vi "PH_BeamlineController.set PA DP Target GUI Elements.vi"(0 "VI in":refnum<vi>, 5 "error in (no error)":errorcluster) -> (14 "VI out":refnum<vi>, 19 "error out":errorcluster)   [LabVIEW 2014, in "PH_BeamlineController.lvlib"]
uses:
  PH_BeamlineController.lvlib
  PH_SystemInformation/PH_SystemInformationEnabling State.ctl
  PH_BeamlineController.Sources.ctl
  PH_SystemInformation/PH_SystemInformation.lvlib
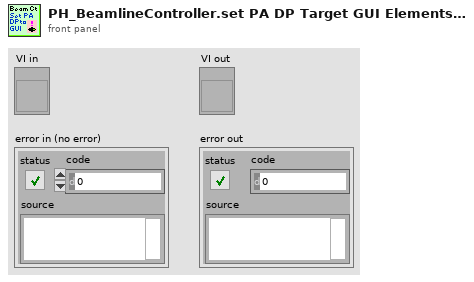
[diagram p1: front panel]
types:
  T1 = typedef "PH_BeamlineController.lvlib/PH_BeamlineController.Sources.ctl" = enum16{"None", "YLF", "fs-Frontend", "ns-Frontend", "YLF and ns-Frontend", "fs- and ns-Frontend"}
  T2 = enum8{"Enabled", "Disabled", "Disabled and Grayed Out"}
  T3 = typedef "PH_SystemInformation.lvlib/PH_SystemInformationEnabling State.ctl" = i32
  T4 = enum16{"Laser", "PreAmp", "MainAmp", "Exp 1", "Exp 2", "Exp 3", "Exp 4"}
  T5 = typedef "PH_BeamlineController.lvlib/PH_BeamlineController.i attribute.ctl" = cluster{"Vacuum Exp LB":cluster{"Channel":string, "Limit [mbar]":dbl, "Pressure [mbar]":dbl, "GUI Ref":refnum<vi>}, "Sources":T6[], "PA DP Targets":T7[], "Path":cluster{"Source":T1, "PA DP Target":T8, "Target":T9}, "Targets":cluster{"Name":T9, "GUI Ref":refnum<vi>, "Current State":bool, "Wanted State":bool, "Enabled":bool}[], "Status Tags":cluster{"Name":string, "Status":T10}[], "special GUI Refs":T11}
  T6 = typedef "PH_BeamlineController.lvlib/PH_BeamlineController.Source Attributes.ctl" = cluster{"Name":T1, "GUI Ref":refnum<vi>, "Current State":bool, "Wanted State":bool}
  T7 = typedef "PH_BeamlineController.lvlib/PH_BeamlineController.PA DP Target Attributes.ctl" = cluster{"Name":T8, "GUI Ref":refnum<vi>, "Current State":bool, "Wanted State":bool, "Enabled":bool}
  T8 = typedef "PH_BeamlineController.lvlib/PH_BeamlineController.PA DP Targets.ctl" = enum16{"None", "Dump PA Delayed Beam", "Dump PA Undelayed Beam", "Dumps PA Delayed and Undelayed Beam"}
  T9 = typedef "PH_BeamlineController.lvlib/PH_BeamlineController.Targets.ctl" = enum16{"None", "PreAmp", "Dump Exp Laserlab", "Exp Laserlab", "Calorimeter", "Dump Exp Laserbay", "Exp Laserbay", "Dump Exp Z6", "Exp Z6"}
  T10 = typedef "PH_StatusHandler.lvlib/PH_StatusHandler.Status.ctl" = i16
  T11 = typedef "PH_BeamlineController.lvlib/PH_BeamlineController.special GUI Refs.ctl" = cluster{"PA-Backreflection-Meas":refnum<vi>, "fs_Synchrolock_Watch":refnum<vi>}
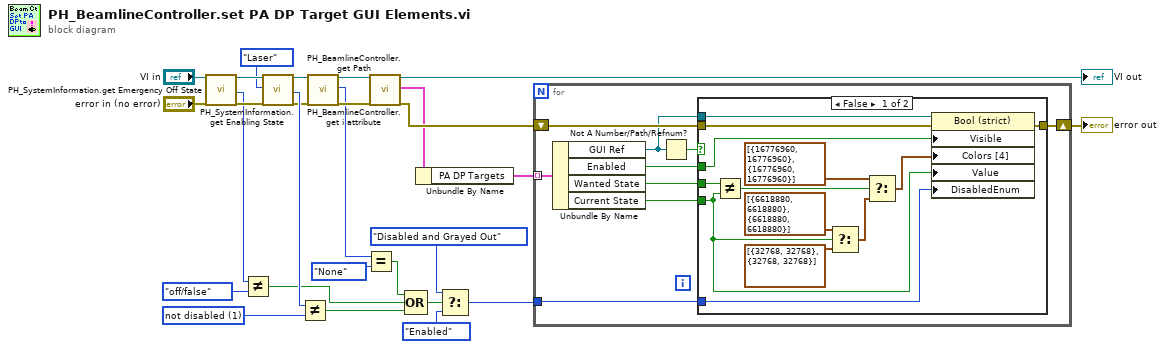
[diagram p0: block diagram]
diagram:
  w16 = T3 1 items=["no info", "not disabled", "disabled"] ("y")
  n1 = call "PH_SystemInformation.get Emergency Off State.vi"("i ref in"="VI in", "error in (no error)"="error in (no error)") -> ("i ref out"=w22:refnum<vi>, "Emergency Off State"=w19:enum16{"no info", "off/false", "Alarm"}, "error out"=w21:errorcluster)  [unwired: 15 in]
  n2 = Not Equal?(x=w19, y=enum16{"no info", "off/false", "Alarm"}."off/false") -> (x != y?=w5:bool)
  n3 = call "PH_SystemInformation.get Enabling State.vi"("i ref in"=w22, "Wanted State"=T4."Laser", "error in (no error)"=w21) -> ("i ref out"=w10:refnum<vi>, "Enabling State"=w17:T3, "error out"=w8:errorcluster)  [unwired: 14 in]
  n4 = Not Equal?(x=w17, y=w16) -> (x != y?=w6:bool)
  n5 = call "PH_BeamlineController.get Path.vi"("VI in"=w10, "error in (no error)"=w8) -> ("VI out"=w9:refnum<vi>, "Path: Source"=w2:T1, "error out"=w7:errorcluster)  [unwired: 12 in, 3 out]
  n6 = Equal?(x=w2, y=PH_BeamlineController.Sources."None" ("Path: Source")) -> (x = y?=w3:bool)
  n7 = call "PH_BeamlineController.get i attribute.vi"("i ref in"=w9, "error in (no error)"=w7) -> ("i ref out"=→"VI out":refnum<vi>, "i attribute"=w24:T5, "error out"=w26:errorcluster)  [unwired: 15 in]
  n8 = Compound Arithmetic op=OR(w3, w5, w6) -> (w4:bool)
  n9 = Unbundle By Name(w24) -> ("PA DP Targets"=w23:T7[])
  n10 = Select(t=T2."Disabled and Grayed Out" ("Disabled"), s=w4, f=T2."Enabled" ("Disabled")) -> (s? t:f=w11:T2)
  n11 = for {
    shift-right: [w35] -> w25
    shift-left: w26 -> [w36]
    tunnel: w23 -> [w34] mode=indexing
    tunnel: w11 -> [w29]
    n12 = Unbundle By Name(w34) -> ("GUI Ref"=w31:refnum<vi>, "Enabled"=w28:bool, "Wanted State"=w33:bool, "Current State"=w32:bool)
    n13 = Not A Number/Path/Refnum?(number/path/refnum=w31) -> (NaN/Path/Refnum?=w30:bool)
    n14 = case shown="False" w30 {
      tunnel: w36 -> [w49 w50]
      tunnel: [w48 w50] -> w35
      tunnel: w31 -> [w47 _]
      tunnel: w33 -> [w41 _]
      tunnel: w32 -> [w40 _]
      tunnel: w29 -> [w39 _]
      tunnel: w28 -> [w37 _]
      frame False {
        n15 = Not Equal?(x=w41, y=w40) -> (x != y?=w44:bool)
        n16 = Select(t=cluster{"Color Box":u32, "Color Box 2":u32}[] [{"Color Box"=6618880, "Color Box 2"=6618880}, {"Color Box"=6618880, "Color Box 2"=6618880}], s=w40, f=cluster{"Color Box":u32, "Color Box 2":u32}[] [{"Color Box"=32768, "Color Box 2"=32768}, {"Color Box"=32768, "Color Box 2"=32768}]) -> (s? t:f=w42:cluster{"Color Box":u32, "Color Box 2":u32}[])
        n17 = Select(t=cluster{"Color Box":u32, "Color Box 2":u32}[] [{"Color Box"=16776960, "Color Box 2"=16776960}, {"Color Box"=16776960, "Color Box 2"=16776960}], s=w44, f=w42) -> (s? t:f=w38:cluster{"Color Box":u32, "Color Box 2":u32}[])
        n18 = property class="Bool (strict)"(reference=w47, error in=w49, "Visible"=w37, "Colors [4]"=w38, "Value"=w40, "DisabledEnum"=w39) -> (error out=w48:errorcluster)  [unwired: 1 out]
      }
      frame True {
      }
    }
  }
  "error out" <- w25
